vi "Get Actual Interface.vi"(8 "error in (no error)":errorcluster, 11 "Output Actor in":refnum<class "Output Actor.lvclass">) -> (0 "error out":errorcluster, 2 "Interface":refnum<class "Output Actor Interface.lvclass">, 3 "Output Actor out":refnum<class "Output Actor.lvclass">)   [LabVIEW 2015, in "Output Actor.lvclass"]
uses:
  Output Actor.lvclass
  Output Actor Interface/Output Actor Interface.lvclass
  Output Actor.lvclass/Output Actor.ctl
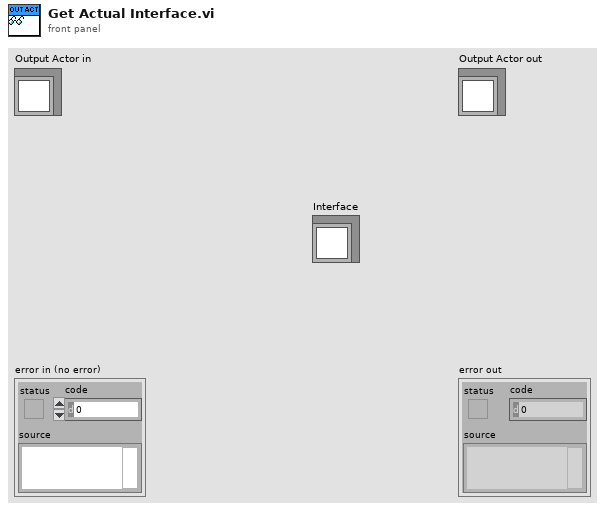
[diagram p1: front panel]
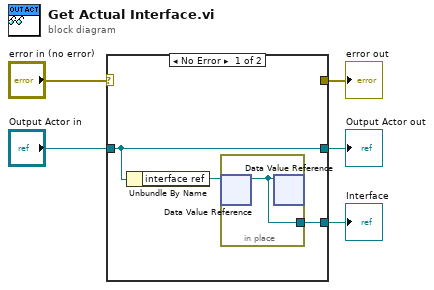
[diagram p0: block diagram]
diagram:
  n1 = case shown="No Error" "error in (no error)" {
    selector: "error in (no error)" -> [_ w10]
    tunnel: [_ w10] -> w4
    tunnel: [w8 w11] -> w2
    tunnel: "Output Actor in" -> [w8 w11]
    tunnel: [w6 _] -> w1
    frame No Error {
      n2 = Unbundle By Name(w8) -> ("interface ref"=w7:refnum<data-value>)
      n3 = in-place {
        in-place-border: [w9] -> w6
        n4 = in-place-dvr #1(w7) -> (w9:refnum<class "Output Actor Interface.lvclass">)  [unwired: 1 out]
        n5 = in-place-dvr #1(w9) -> ()  [unwired: 2 out]
      }
    }
    frame Error {
    }
  }
  "error out" <- w4
  "Output Actor out" <- w2
  "Interface" <- w1
